vi "Pre Launch Init.vi"(11 "Event Source In":refnum<class "Event Source.lvclass">) -> (0 "Error Out":errorcluster, 3 "Event Source Out":refnum<class "Event Source.lvclass">)   [LabVIEW 2016, in "Event Source.lvlib" / "Event Source.lvclass"]
doc: "(<B>Filename</B>: Actor Framework.lvlib:Actor.lvclass:Pre Launch Init.vi)\n\nDefines behavior that occurs after the Launch Nested Actor method is invoked but before the actor's Actor Core method begins running.\n\nBy default, this method does nothing. A descendant class may override it to define behavior."
uses:
  Event Source.lvclass
  Event Source.lvclass/Event Source.ctl
  <vilib>/MGI/Monitored Actor/Monitored Actor/Monitored Actor/Monitored Actor.lvclass
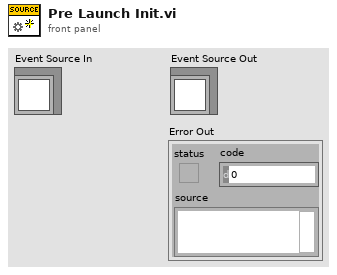
[diagram p1: front panel]
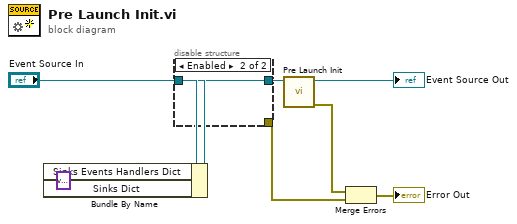
[diagram p0: block diagram]
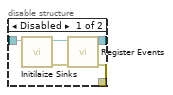
[diagram p2: hidden frame]
diagram:
  w1 = variant ("Events Dict")
  n1 = Bundle By Name(cluster="Event Source In", "Sinks Events Handlers Dict"=w1, "Sinks Dict"=w1) -> (w2:refnum<class "Event Source.lvclass">)
  n2 = disable-structure shown="Enabled" {
    disable-tunnel: [w13 w14] -> w4
    disable-tunnel: [w12 _] -> w3
    disable-tunnel: w2 -> [w9 w14]
    frame Disabled {
      n3 = call-dynamic "Initilaize Sinks.vi"("Event Source in"=w9) -> ("error out"=w11:errorcluster, "Event Source out"=w10:refnum<class "Event Source.lvclass">)  [unwired: 9 in]
      n4 = call-dynamic "Register Events.vi"("error in (no error)"=w11, "Event Source in"=w10) -> ("error out"=w12:errorcluster, "Event Source out"=w13:refnum<class "Event Source.lvclass">)  [unwired: 8 in]
    }
    frame Enabled {
    }
  }
  n5 = call-parent "Pre Launch Init.vi"("Monitored Actor in"=w4) -> ("error out"=w6:errorcluster, "Monitored Actor out"=→"Event Source Out":refnum<class "Event Source.lvclass">)  [unwired: 9 in]
  n6 = Merge Errors(w6, w3) -> (→"Error Out":errorcluster)
